vi "elapsed_sec_test.vi"() -> ()   [LabVIEW 2015]
uses:
  BERTTA.dll
panel:
  out "element 4":i32
  in  "reset":i32
  out "element 3":i32
  in  "enable":i32
  out "element 2":i32
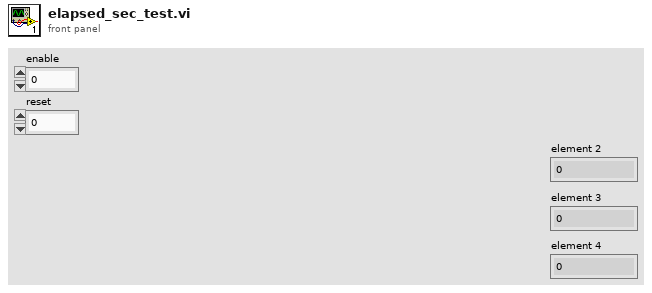
[diagram p1: front panel]
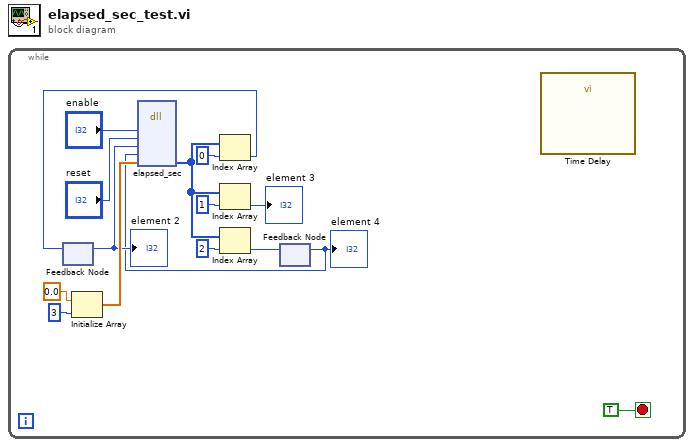
[diagram p0: block diagram]
diagram:
  n1 = while {
    stop <- TRUE stop-if-true
    n2 = feedback #1() -> (w3:i32)  [unwired: 1 in]
    "element 2" <- w3
    n3 = Initialize Array(0.0 ("element"), 3 ("dimension size")) -> (w12:dbl[])
    n4 = feedback #2() -> (w1:i32)  [unwired: 1 in]
    "element 4" <- w1
    n5 = dll-call lib="C:/Users/shresplab/OneDrive - Kemira Oyj/Documents/Visual Studio 2017/Projects/Bertta/BERTTA/x64/Debug/BERTTA.dll" fn="elapsed_sec"("enable"="enable", "reset"="reset", "last_time"=w3, "elapsed_last"=w1, "params"=w12) -> ("params"=w6:i32[])  [unwired: 8 in, 2 out]
    n6 = Index Array(array=w6, index=0) -> (element=w4:i32)
    n7 = feedback-in #1(w4) -> ()
    n8 = Index Array(array=w6, index=1) -> (element=→"element 3":i32)
    n9 = Index Array(array=w6, index=2) -> (element=w2:i32)
    n10 = feedback-in #2(w2) -> ()
    n11 = call "Time Delay"() -> ()  [unwired: 11 in, 1 out]
  }
